vi "setTiming.vi"(8 "error in (no error)":errorcluster, 11 "DIO64Output in":refnum<class "DIO64Output.lvclass">) -> (0 "error out":errorcluster, 3 "DIO64Output out":refnum<class "DIO64Output.lvclass">)   [LabVIEW 2011, in "Hardware.lvlib" / "Channels.lvlib" / "DIO64Output.lvclass"]
uses:
  DIO64Output.lvclass
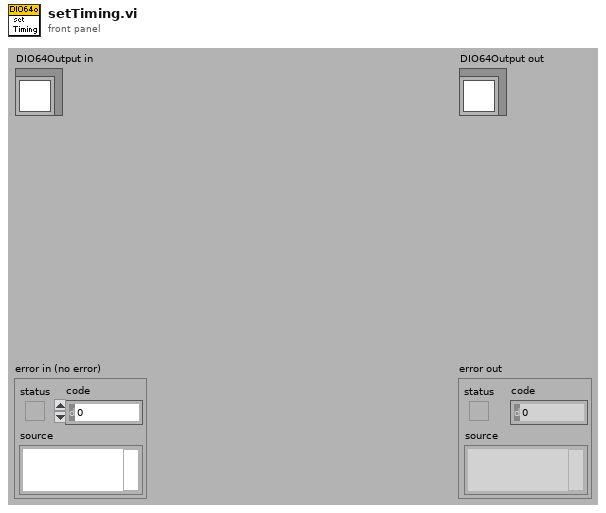
[diagram p1: front panel]
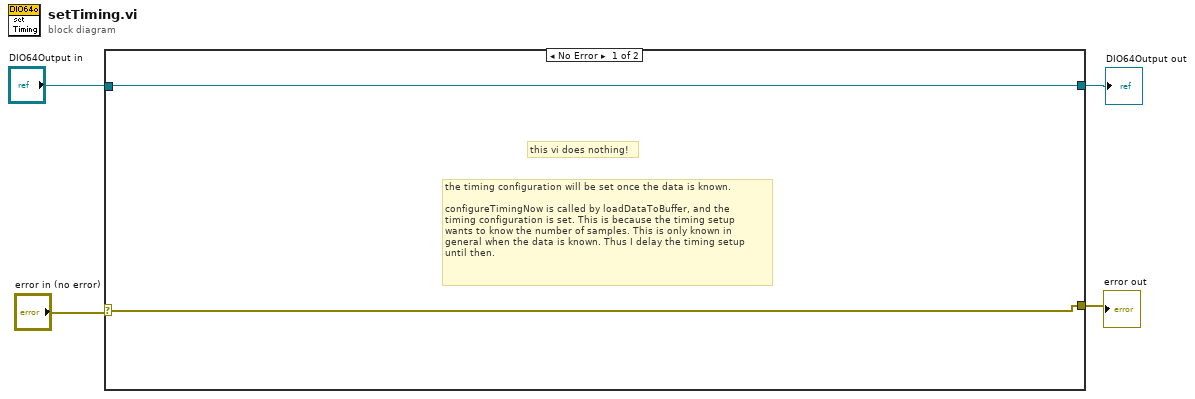
[diagram p0: block diagram]
diagram:
  n1 = case shown="No Error" "error in (no error)" {
    selector: "error in (no error)" -> [w6 w7]
    tunnel: "DIO64Output in" -> [w5 w8]
    tunnel: [w5 w8] -> w2
    tunnel: [w6 w7] -> w1
    frame No Error {
      # "the timing configuration will be set once the data is known.\n\nconfigureTimingNow is called by loadDataToBuffer, and the\ntiming configuration is set. This is because the timing setup\nwants to know the number of samples. This is only known in\ngeneral when the data is known. Thus I delay the timing setup\nuntil then."
      # "this vi does nothing!"
    }
    frame Error {
    }
  }
  "error out" <- w1
  "DIO64Output out" <- w2
